vi "Create IO Config Table.vi"(8 "error in (no error)":errorcluster, 10 "connection reference":T1, 11 "Table in":refnum<vi>) -> (0 "error out":errorcluster)   [LabVIEW 2018]
uses:
  <vilib>/addons/database/Connection.llb/Conn ObjectReference.ctl
  <vilib>/addons/database/Auxilliary.llb/DB Tools Column Info.ctl
  <vilib>/addons/database/Auxilliary.llb/DB Tools DataTypes.ctl
  <vilib>/addons/database/NI_Database_API.lvlib
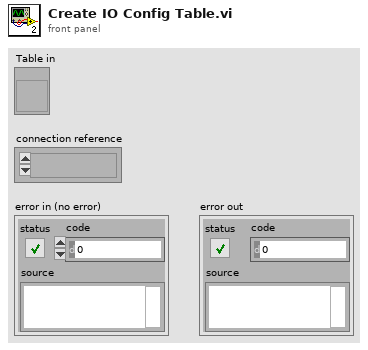
[diagram p1: front panel]
types:
  T1 = typedef "NI_Database_API.lvlib/Conn ObjectReference.ctl" = refnum<k1>
  T2 = typedef "NI_Database_API.lvlib/DB Tools Column Info.ctl" = cluster{"column name":string, "data type":T3, "size":i32, "allow null?":bool}
  T3 = typedef "NI_Database_API.lvlib/DB Tools DataTypes.ctl" = enum16{"String", "Long (I32)", "Single (SGL)", "Double (DBL)", "Date/Time", "Binary"}
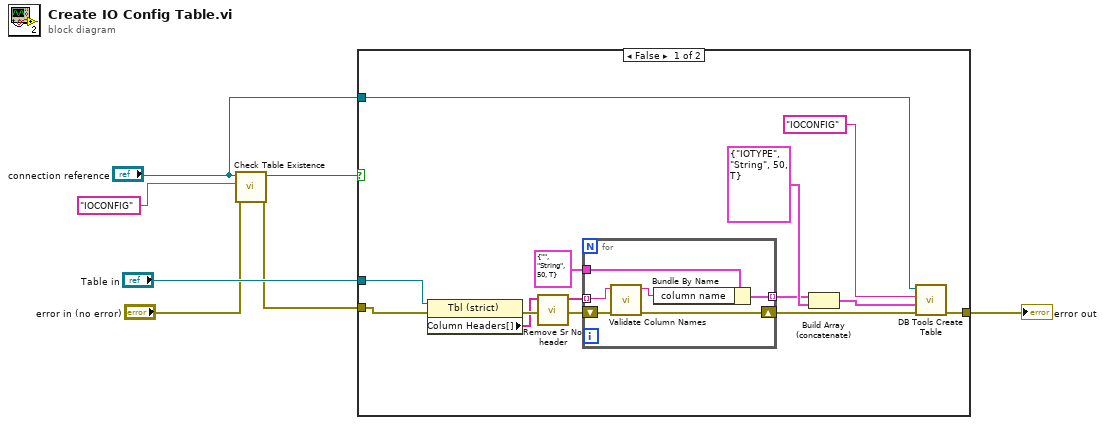
[diagram p0: block diagram]
diagram:
  n1 = call "Check Table Existence.vi"("error in (no error)"="error in (no error)", "element"="IOCONFIG", "Refnum in"="connection reference") -> ("error out"=w3:errorcluster, "Table Exist?"=w2:bool)  [unwired: 7 in]
  n2 = case shown="False" w2 {
    tunnel: [w18 w27] -> w7
    tunnel: "Table in" -> [w10 _]
    tunnel: w3 -> [w9 w27]
    tunnel: "connection reference" -> [w8 _]
    frame False {
      n3 = property on="Property Node" class="Tbl (strict)"(reference=w10, error in=w9) -> (error out=w20:errorcluster, "Column Headers[]"=w11:string[])  [unwired: 1 out]
      n4 = call "Remove Sr No header.vi"("Column Headers[] in"=w11) -> ("Column Headers[] out"=w13:string[])  [unwired: 10 in]
      n5 = for {
        tunnel: T2 {"column name"="", "data type"=enum."String", "size"=50, "allow null?"=TRUE} ("column information") -> [w26]
        tunnel: w13 -> [w24] mode=indexing
        tunnel: [w25] -> w14 mode=indexing
        shift-right: [w22] -> w19
        shift-left: w20 -> [w21]
        n6 = call "Validate Column Names.vi"("error in (no error)"=w21, "Label.Text"=w24) -> ("error out"=w22:errorcluster, "result string"=w23:string)  [unwired: 8 in]
        n7 = Bundle By Name(cluster=w26, "column name"=w23) -> (w25:T2)
      }
      n8 = Build Array (concatenate)(w14, T2 {"column name"="IOTYPE", "data type"=enum."String", "size"=50, "allow null?"=TRUE} ("column information")) -> (w16:T2[])
      n9 = call <vilib>:"DB Tools Create Table.vi"("error in (no error)"=w19, "column information"=w16, "table"="IOCONFIG", "connection reference"=w8) -> ("error out"=w18:errorcluster)  [unwired: 4 in, 1 out]
    }
    frame True {
    }
  }
  "error out" <- w7
